vi "svx_Orbit Facade.vi"(0 "Data In":T5, 2 "Display State In":T3, 3 "Container State":T4) -> (6 "Data Out":T5, 7 "Display State Out":T3, 8 "Action":T2)   [LabVIEW 2017, in "SVX Orbit.xctl"]
uses:
  <vilib>/addons/_XControls/Orbit Plot/SVX Orbit.xctl
  <vilib>/addons/_XControls/Orbit Plot/subVIs/svx_Orbit Data.ctl
  <vilib>/_xctls/Container State.ctl
  <vilib>/addons/_XControls/Orbit Plot/subVIs/svx_Orbit State.ctl
  <vilib>/addons/_XControls/Orbit Plot/subVIs/svx_Orbit Internal State.ctl
  <vilib>/addons/_XControls/Orbit Plot/subVIs/svx_Orbit Bounds.ctl
  <vilib>/_xctls/Action.ctl
  <vilib>/Utility/miscctls.llb/LVPoint32TypeDef.ctl
  <vilib>/addons/_XControls/Orbit Plot/subVIs/svx_Orbit Core States.ctl
  <vilib>/_xctls/XControlSupport.lvlib
panel:
  out "Coords":T1
  out "Tree":string(tree)
  out "Cursor Info":string
  out "Orbit Plot":T6(graph)=[{"orbit plot X"=[1.0], "orbit plot Y"=[1.0]}, {"orbit plot X"=[0.0, 1.0], "orbit plot Y"=[1.0]}]
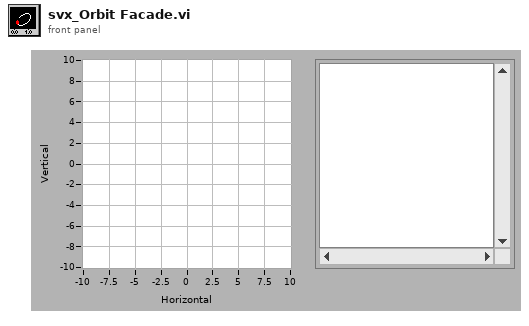
[diagram p1: front panel]
types:
  T1 = typedef "LVPoint32TypeDef.ctl" = cluster{"Horizontal":i32, "Vertical":i32}
  T2 = typedef "XControlSupport.lvlib/Action.ctl" = cluster{"Data Changed?":bool, "State Changed?":bool, "Action Name":string}
  T3 = typedef "SVX Orbit.xctl/svx_Orbit State.ctl" = cluster{"State Queue":refnum<queue>, "Old State":variant}
  T4 = typedef "XControlSupport.lvlib/Container State.ctl" = cluster{"Indicator?":bool, "Run Mode?":bool, " Refnum":refnum<vi>}
  T5 = typedef "SVX Orbit.xctl/svx_Orbit Data.ctl" = cluster{"probe x":dbl[], "probe y":dbl[], "reference":dbl[], "plot type":enum16{"Filtered Plot", "Unfiltered Plot"}, "attribute":variant}[][]
  T6 = cluster{"orbit plot X":dbl[], "orbit plot Y":dbl[]}[]
  T7 = cluster{"CursLoc.X":dbl, "Cursloc.Y":dbl, "PointIdx":i32}
  T8 = cluster{"Minimum":dbl, "Maximum":dbl, "Kind":enum16{"X-Scale", "Y-Scale", "Z-Scale"}}
  T9 = typedef "SVX Orbit.xctl/svx_Orbit Internal State.ctl" = cluster{"X Scale":cluster{"Name":string, "FString":string, "Major Color":u32, "Minor Color":u32, "Scale Visible":bool, " Label Visible":bool, "Grid Style":u16}, "Y Scale":cluster{"Name":string, "FString":string, "Major Color":u32, "Minor Color":u32, "Scale Visible":bool, " Label Visible":bool, "Grid Style":u16}, "Plot":cluster{"Point Style":u8, "Line Width":u8, "Line Style":u8, "Plot Color":u32, "Point/fill":u32}, "Arrow/Crosshair Color":u32, "Tacho Point Color":u32, "Container Bounds":T10, "Axis Maximum":dbl, "Probe Angles":cluster{"Angle X":dbl, "Angle Y":dbl}, "Background Color":u32, "Cursor":cluster{"Cursor Point Style":u8, "Cursor Style":u8, "Cursor Line Width":u8, "Cursor Line Style":u8, "Cursor Color":u32, "Cursor Name Visible":bool, "Cursor Visible":bool, "Cursor Position":cluster{"X":dbl, "Y":dbl}, "Cursor Index":i32, "Cursor Lock":bool}, "Elliptical Info":cluster{"a":dbl, "b":dbl, "e":dbl, "ang":dbl}[], "Legend Visible":bool, "Scale Range Change":refnum<user-event>, "Strings[]":cluster{"Custom pair name":bool, "Row Strings []":string[], "Column Strings []":string[]}, "Index":cluster{"pair index":i32, "order index":i32}[], " Parents Tags":string[], "Children Tags":string[], "Open?":bool[], "Label":string, "Legend Width":u32, "Pair Strings Changed?":bool, "Size":i32[], "Legend Background":u32, "Legend Font":u32, "Cursor Release":refnum<user-event>, "Autoscale":bool, "Precession Direction":enum16{"forward", "backward"}[], "Item Width":u32, "User Pair Strings []":string[], "Users Order Strings []":string[], "Autoscale Once":bool, "Property Write":refnum<queue>}
  T10 = typedef "SVX Orbit.xctl/svx_Orbit Bounds.ctl" = cluster{"Width":u32, "Height":u32}
  T11 = typedef "SVX Orbit.xctl/svx_Orbit Core States.ctl" = enum16{"None", "[Axis] Range", "[Plot] Image", "[Plot] Tacho Point", "[Plot] Grid and BG", "[Cursor] Cursor Info", "[Legend] Pair Strings", "[Data] Plot Data", "[Legend] Checkbox", "[Layout] Update", "[Legend] Tree Open", "[Layout] Legend Visible", "[Plot] Data Point", "[Axis] Axis and Label", "[Axis] Format String", "[Cursor] Appearance", "[Cursor] Index", "[Legend] Color", "[Layout] Min Pane Size", "[Data] Legend Strings"}
  T12 = typedef "LVRangeTypeDef.ctl" = cluster{"Minimum":dbl, "Maximum":dbl, "Increment":dbl, "Minor Increment":dbl, "Start":dbl}
  T13 = cluster{" Refnum":refnum<vi>, "Orbit Plot":refnum<vi>, "Tree":refnum<vi>, "Cursor Info":refnum<vi>, "This VI":refnum<vi>}
  T14 = cluster{"BG Color":u32, "XScale.MajGrdColor":u32, "XScale.MnrGrdColor":u32, "YScale.MajGrdColor":u32, "YScale.MnrGrdColor":u32}
  T15 = cluster{"Background Color":u32, "Major Color":u32, "Minor Color":u32, "Major Color":u32, "Minor Color":u32}
  T16 = typedef "LVRectTypeDef.ctl" = cluster{"Left":i16, "Top":i16, "Right":i16, "Bottom":i16}
  T17 = cluster{"Shift":bool, "Ctrl":bool, "Alt":bool, "Cmd":bool, "Opt":bool}
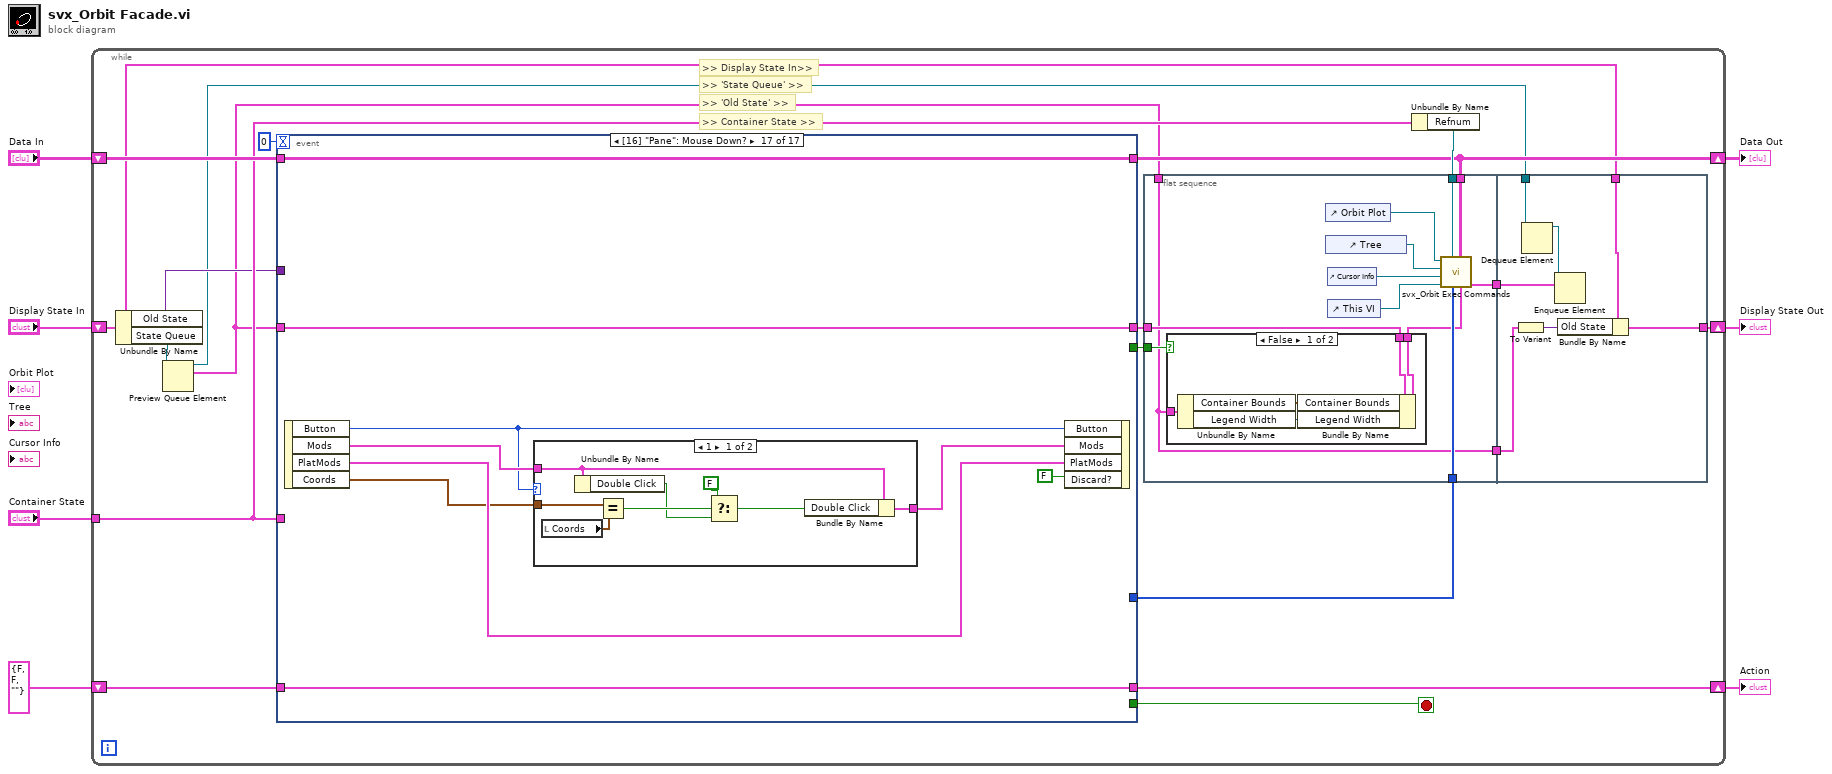
[diagram p0: block diagram]
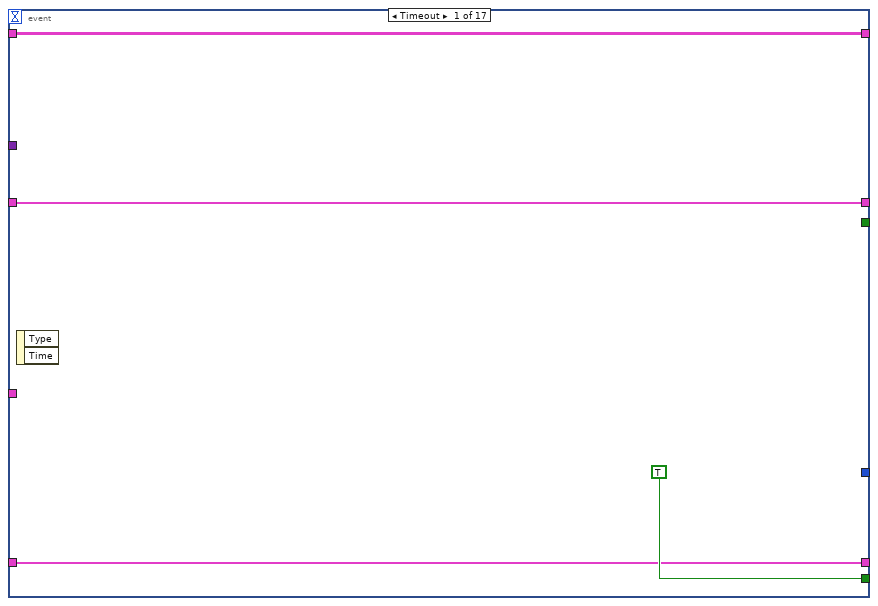
[diagram p3: hidden frame]
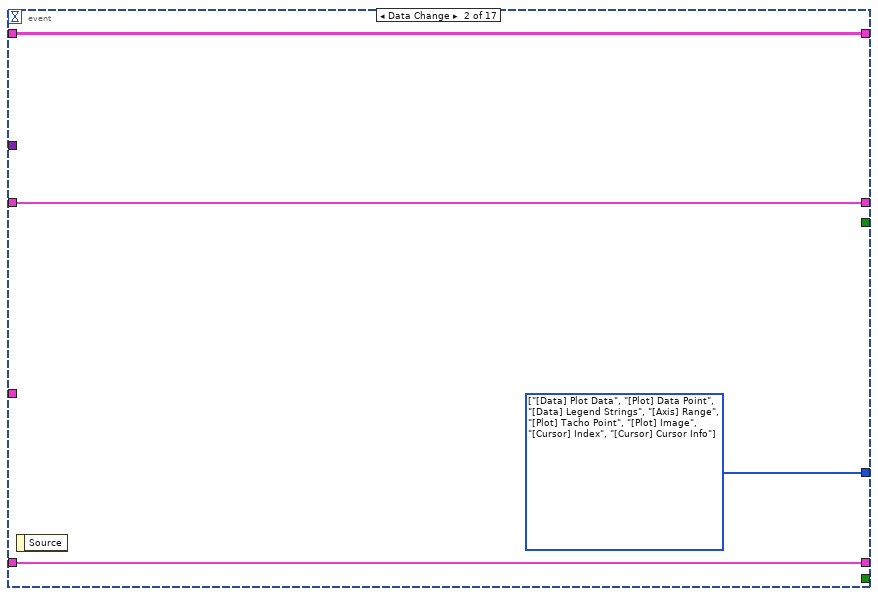
[diagram p4: hidden frame]
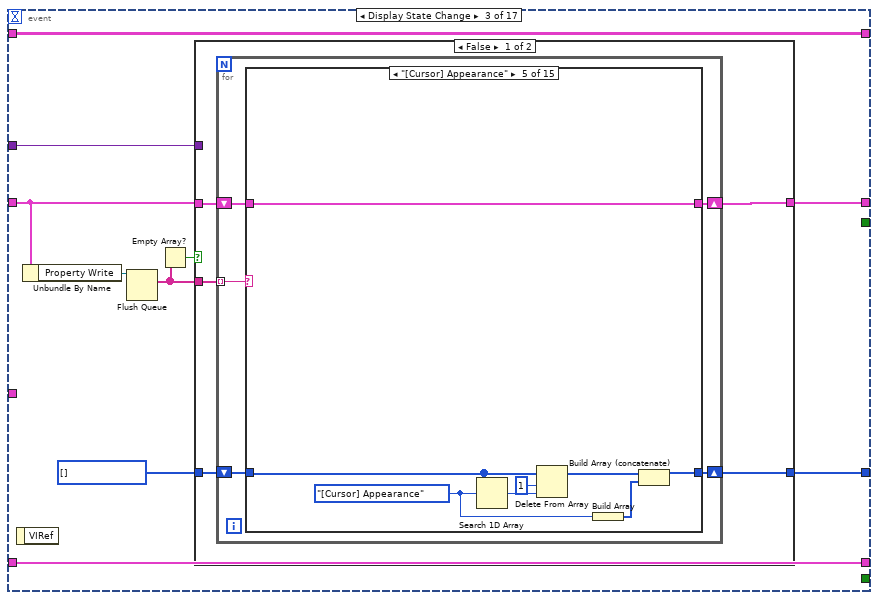
[diagram p5: hidden frame]
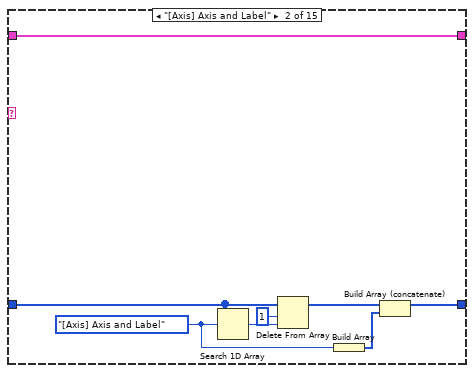
[diagram p7: hidden frame]
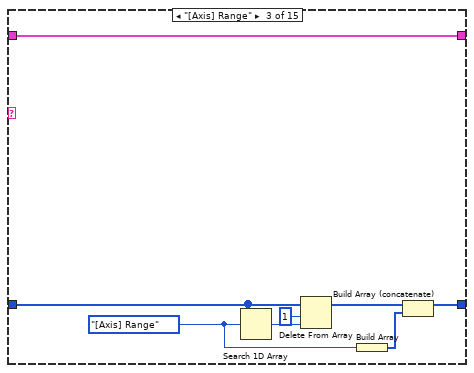
[diagram p8: hidden frame]
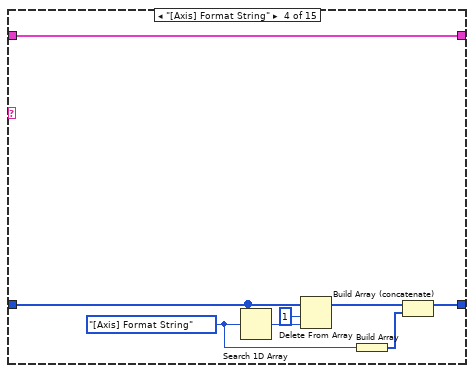
[diagram p9: hidden frame]
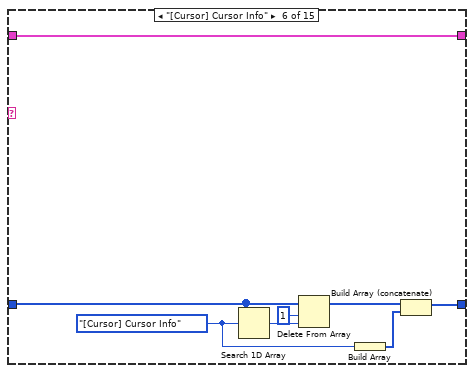
[diagram p10: hidden frame]
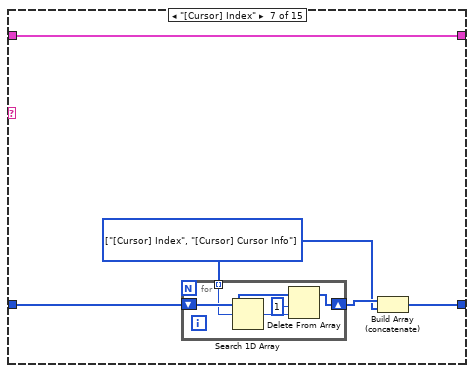
[diagram p11: hidden frame]
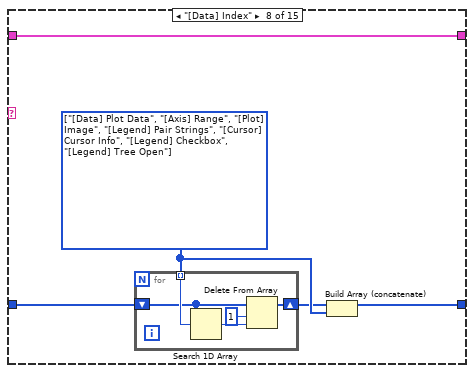
[diagram p12: hidden frame]
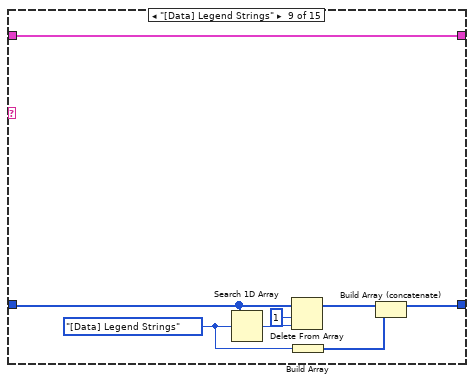
[diagram p13: hidden frame]
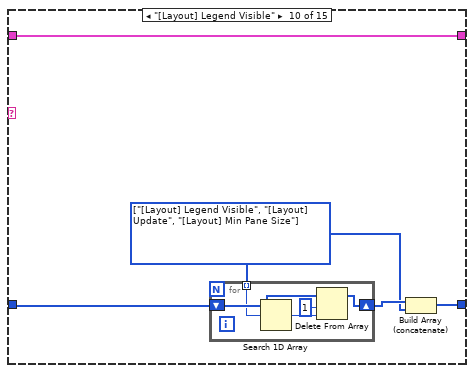
[diagram p14: hidden frame]
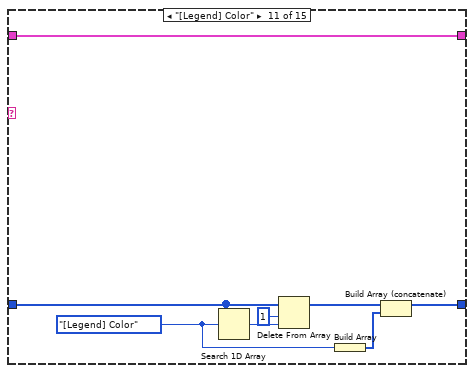
[diagram p15: hidden frame]
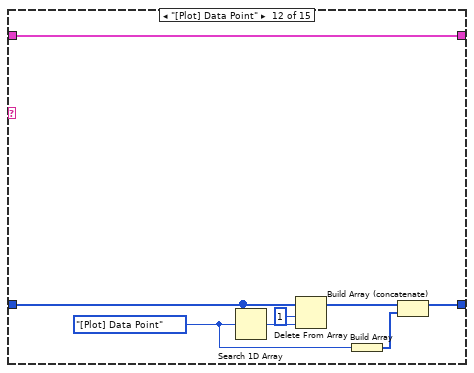
[diagram p16: hidden frame]
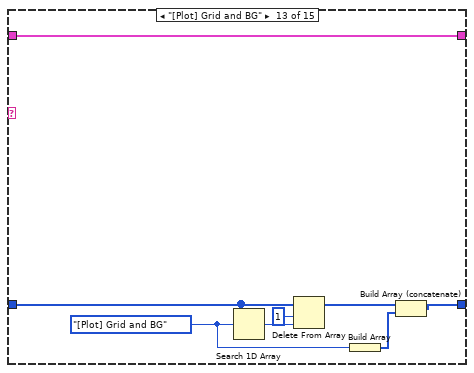
[diagram p17: hidden frame]
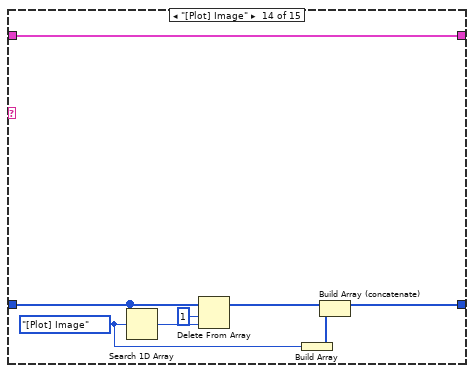
[diagram p18: hidden frame]
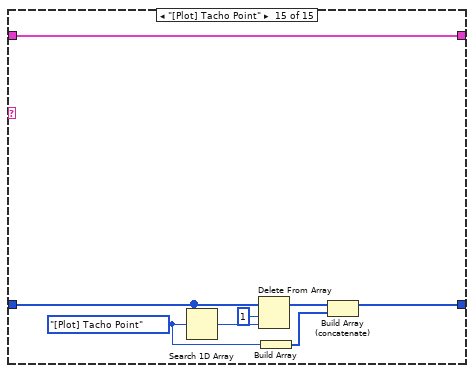
[diagram p19: hidden frame]
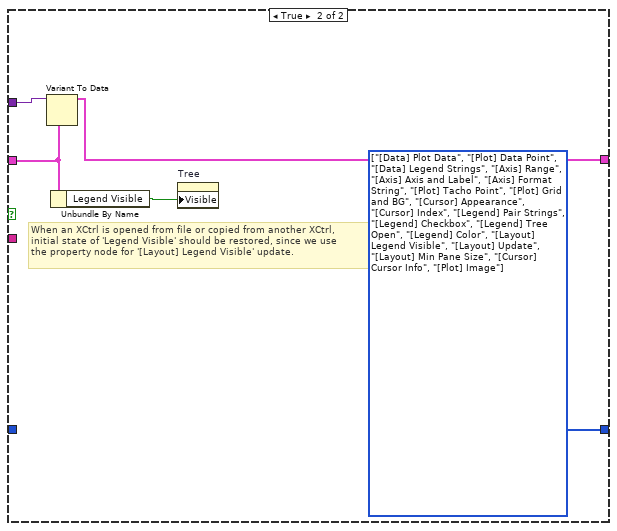
[diagram p20: hidden frame]
diagram:
  n1 = while {
    shift-right: [w11] -> w4
    shift-left: "Display State In" -> [w12]
    tunnel: "Container State" -> [w23]
    shift-right: [w21] -> w7
    shift-left: "Data In" -> [w25]
    shift-right: [w18] -> w2
    shift-left: T2 {"Data Changed?"=FALSE, "State Changed?"=FALSE, "Action Name"=""} ("Action") -> [w24]
    stop <- w16 stop-if-true
    # ">> Container State >>"
    # ">> 'Old State' >>"
    # ">> Display State In>>"
    # ">> 'State Queue' >>"
    n2 = Unbundle By Name(w12) -> ("Old State"=w15:variant, "State Queue"=w17:refnum<queue>)
    n3 = Preview Queue Element(queue=w17) -> (queue out=w13:refnum<queue>, element=w9:T9)  [unwired: 2 in, 2 out]
    n4 = event shown="[16] \"Pane\": Mouse Down?" {
      selector: _ -> [_ _ _ _ _ _ _ _ _ _ _ _ _ _ _ _ _]
      dyn-events: _ -> [_ _ _ _ _ _ _ _ _ _ _ _ _ _ _ _ _]
      timeout: 0 -> [_ _ _ _ _ _ _ _ _ _ _ _ _ _ _ _ _]
      tunnel: w9 -> [w52 w58 w60 w207 w210 w222 w256 w277 w288 w298 w397 w480 w510 w518 w557 w562 w581]
      tunnel: [w52 w58 w66 w207 w210 w214 w228 w280 w288 w297 w396 w479 w509 w521 w557 w562 w581] -> w20
      tunnel: [TRUE _ _ _ _ _ _ _ _ _ _ _ _ _ _ _ _] -> w16
      tunnel: w23 -> [_ _ _ _ _ _ _ _ w292 w303 _ _ _ _ _ _ _]
      tunnel: w25 -> [w54 w59 w65 w206 w209 w221 w261 w286 w294 w295 w400 w482 w504 w528 w555 w561 w582]
      tunnel: [w54 w59 w65 w206 w209 w221 w261 w286 w294 w295 w400 w481 w504 w528 w555 w561 w582] -> w21
      tunnel: [w53 w56 w64 w205 w208 w224 w259 w276 w293 w296 w394 w485 w507 w519 w556 w560 w580] -> w18
      tunnel: w24 -> [w53 w56 w64 w205 w208 w225 w260 w276 w293 w300 w395 w487 w508 w520 w556 w560 w580]
      tunnel: [_ w57 w68 _ _ w219 _ w285 _ w299 w393 w486 _ w517 _ _ _] -> w19
      tunnel: w15 -> [_ _ w63 _ _ _ _ _ _ _ _ _ _ _ _ _ _]
      tunnel: [_ _ _ _ _ _ _ TRUE _ _ _ _ _ _ _ _ _] -> w10
      event Timeout {
        n5 = event-data() -> ()  [unwired: 1 in, 2 out]
      }
      event Data Change {
        w57 = T11[] [enum."[Data] Plot Data", enum."[Plot] Data Point", enum."[Data] Legend Strings", enum."[Axis] Range", enum."[Plot] Tacho Point", enum."[Plot] Image", enum."[Cursor] Index", enum."[Cursor] Cursor Info"] items=["None", "[Axis] Range", "[Plot] Image", "[Plot] Tacho Point", "[Plot] Grid and BG", "[Cursor] Cursor Info", "[Legend] Pair Strings", "[Data] Plot Data", "[Legend] Checkbox", "[Layout] Update", "[Legend] Tree Open", "[Layout] Legend Visible", "[Plot] Data Point", "[Axis] Axis and Label", "[Axis] Format String", "[Cursor] Appearance", "[Cursor] Index", "[Legend] Color", "[Layout] Min Pane Size", "[Data] Legend Strings"] ("array")
        n6 = event-data() -> ()  [unwired: 1 in, 1 out]
      }
      event Display State Change {
        w67 = T11[] [] items=["None", "[Axis] Range", "[Plot] Image", "[Plot] Tacho Point", "[Plot] Grid and BG", "[Cursor] Cursor Info", "[Legend] Pair Strings", "[Data] Plot Data", "[Legend] Checkbox", "[Layout] Update", "[Legend] Tree Open", "[Layout] Legend Visible", "[Plot] Data Point", "[Axis] Axis and Label", "[Axis] Format String", "[Cursor] Appearance", "[Cursor] Index", "[Legend] Color", "[Layout] Min Pane Size", "[Data] Legend Strings"]
        n7 = event-data() -> ()  [unwired: 1 in, 1 out]
        n8 = Unbundle By Name(w60) -> ("Property Write"=w62:refnum<queue>)
        n9 = Flush Queue(queue=w62) -> (remaining elements=w61:string[])  [unwired: 1 in, 2 out]
        n10 = Empty Array?(array=w61) -> (empty?=w69:bool)
        n11 = case shown="False" w69 {
          tunnel: w60 -> [w72 w201]
          tunnel: [w73 w204] -> w68
          tunnel: w67 -> [w74 _]
          tunnel: [w71 w200] -> w66
          tunnel: w63 -> [_ w203]
          tunnel: w61 -> [w70 _]
          frame False {
            n12 = for {
              tunnel: w70 -> [w79] mode=indexing
              shift-right: [w77] -> w73
              shift-left: w74 -> [w78]
              shift-right: [w75] -> w71
              shift-left: w72 -> [w76]
              n13 = case shown="\"[Cursor] Appearance\"" w79 {
                tunnel: w78 -> [w81 w83 w91 w99 w107 w115 w124 w135 w144 w151 w161 w169 w178 w187 w195]
                tunnel: [w81 w82 w90 w98 w106 w114 w123 w132 w143 w150 w160 w168 w177 w191 w199] -> w77
                tunnel: w76 -> [w80 w89 w97 w105 w113 w121 w126 w136 w149 w154 w167 w175 w183 w190 w198]
                tunnel: [w80 w89 w97 w105 w113 w121 w126 w136 w149 w154 w167 w175 w183 w190 w198] -> w75
                frame "", Default {
                }
                frame "[Axis] Axis and Label" {
                  w84 = svx_Orbit_Core_States."[Axis] Axis and Label" ("Property Page User Events")
                  n14 = Search 1D Array(1D array=w83, element=w84) -> (index of element=w88:i32)  [unwired: 1 in]
                  n15 = Delete From Array(array=w83, length=1, index=w88) -> (array with subset deleted=w86:T11[])  [unwired: 1 out]
                  n16 = Build Array(w84) -> (w85:T11[])
                  n17 = Build Array (concatenate)(w86, w85) -> (w82:T11[])
                }
                frame "[Axis] Range" {
                  w92 = svx_Orbit_Core_States."[Axis] Range" ("Property Page User Events")
                  n18 = Search 1D Array(1D array=w91, element=w92) -> (index of element=w96:i32)  [unwired: 1 in]
                  n19 = Delete From Array(array=w91, length=1, index=w96) -> (array with subset deleted=w94:T11[])  [unwired: 1 out]
                  n20 = Build Array(w92) -> (w93:T11[])
                  n21 = Build Array (concatenate)(w94, w93) -> (w90:T11[])
                }
                frame "[Axis] Format String" {
                  w100 = svx_Orbit_Core_States."[Axis] Format String" ("Property Page User Events")
                  n22 = Search 1D Array(1D array=w99, element=w100) -> (index of element=w104:i32)  [unwired: 1 in]
                  n23 = Delete From Array(array=w99, length=1, index=w104) -> (array with subset deleted=w102:T11[])  [unwired: 1 out]
                  n24 = Build Array(w100) -> (w101:T11[])
                  n25 = Build Array (concatenate)(w102, w101) -> (w98:T11[])
                }
                frame "[Cursor] Appearance" {
                  w109 = svx_Orbit_Core_States."[Cursor] Appearance" ("Property Page User Events")
                  n26 = Search 1D Array(1D array=w107, element=w109) -> (index of element=w112:i32)  [unwired: 1 in]
                  n27 = Delete From Array(array=w107, length=1, index=w112) -> (array with subset deleted=w108:T11[])  [unwired: 1 out]
                  n28 = Build Array(w109) -> (w110:T11[])
                  n29 = Build Array (concatenate)(w108, w110) -> (w106:T11[])
                }
                frame "[Cursor] Cursor Info" {
                  w117 = svx_Orbit_Core_States."[Cursor] Cursor Info" ("Property Page User Events")
                  n30 = Search 1D Array(1D array=w115, element=w117) -> (index of element=w120:i32)  [unwired: 1 in]
                  n31 = Delete From Array(array=w115, length=1, index=w120) -> (array with subset deleted=w116:T11[])  [unwired: 1 out]
                  n32 = Build Array(w117) -> (w118:T11[])
                  n33 = Build Array (concatenate)(w116, w118) -> (w114:T11[])
                }
                frame "[Cursor] Index" {
                  w122 = T11[] [enum."[Cursor] Index", enum."[Cursor] Cursor Info"] items=["None", "[Axis] Range", "[Plot] Image", "[Plot] Tacho Point", "[Plot] Grid and BG", "[Cursor] Cursor Info", "[Legend] Pair Strings", "[Data] Plot Data", "[Legend] Checkbox", "[Layout] Update", "[Legend] Tree Open", "[Layout] Legend Visible", "[Plot] Data Point", "[Axis] Axis and Label", "[Axis] Format String", "[Cursor] Appearance", "[Cursor] Index", "[Legend] Color", "[Layout] Min Pane Size", "[Data] Legend Strings"]
                  n34 = for {
                    shift-right: [w128] -> w125
                    shift-left: w124 -> [w129]
                    tunnel: w122 -> [w127] mode=indexing
                    n35 = Search 1D Array(1D array=w129, element=w127) -> (index of element=w131:i32)  [unwired: 1 in]
                    n36 = Delete From Array(array=w129, length=1, index=w131) -> (array with subset deleted=w128:T11[])  [unwired: 1 out]
                  }
                  n37 = Build Array (concatenate)(w125, w122) -> (w123:T11[])
                }
                frame "[Data] Index" {
                  w134 = T11[] [enum."[Data] Plot Data", enum."[Axis] Range", enum."[Plot] Image", enum."[Legend] Pair Strings", enum."[Cursor] Cursor Info", enum."[Legend] Checkbox", enum."[Legend] Tree Open"] items=["None", "[Axis] Range", "[Plot] Image", "[Plot] Tacho Point", "[Plot] Grid and BG", "[Cursor] Cursor Info", "[Legend] Pair Strings", "[Data] Plot Data", "[Legend] Checkbox", "[Layout] Update", "[Legend] Tree Open", "[Layout] Legend Visible", "[Plot] Data Point", "[Axis] Axis and Label", "[Axis] Format String", "[Cursor] Appearance", "[Cursor] Index", "[Legend] Color", "[Layout] Min Pane Size", "[Data] Legend Strings"]
                  n38 = for {
                    tunnel: w134 -> [w139] mode=indexing
                    shift-right: [w137] -> w133
                    shift-left: w135 -> [w138]
                    n39 = Search 1D Array(1D array=w138, element=w139) -> (index of element=w141:i32)  [unwired: 1 in]
                    n40 = Delete From Array(array=w138, length=1, index=w141) -> (array with subset deleted=w137:T11[])  [unwired: 1 out]
                  }
                  n41 = Build Array (concatenate)(w133, w134) -> (w132:T11[])
                }
                frame "[Data] Legend Strings" {
                  w142 = svx_Orbit_Core_States."[Data] Legend Strings" ("Property Page User Events")
                  n42 = Search 1D Array(1D array=w144, element=w142) -> (index of element=w148:i32)  [unwired: 1 in]
                  n43 = Delete From Array(array=w144, length=1, index=w148) -> (array with subset deleted=w146:T11[])  [unwired: 1 out]
                  n44 = Build Array(w142) -> (w145:T11[])
                  n45 = Build Array (concatenate)(w146, w145) -> (w143:T11[])
                }
                frame "[Layout] Legend Visible" {
                  w152 = T11[] [enum."[Layout] Legend Visible", enum."[Layout] Update", enum."[Layout] Min Pane Size"] items=["None", "[Axis] Range", "[Plot] Image", "[Plot] Tacho Point", "[Plot] Grid and BG", "[Cursor] Cursor Info", "[Legend] Pair Strings", "[Data] Plot Data", "[Legend] Checkbox", "[Layout] Update", "[Legend] Tree Open", "[Layout] Legend Visible", "[Plot] Data Point", "[Axis] Axis and Label", "[Axis] Format String", "[Cursor] Appearance", "[Cursor] Index", "[Legend] Color", "[Layout] Min Pane Size", "[Data] Legend Strings"]
                  n46 = for {
                    shift-right: [w156] -> w153
                    shift-left: w151 -> [w157]
                    tunnel: w152 -> [w155] mode=indexing
                    n47 = Search 1D Array(1D array=w157, element=w155) -> (index of element=w159:i32)  [unwired: 1 in]
                    n48 = Delete From Array(array=w157, length=1, index=w159) -> (array with subset deleted=w156:T11[])  [unwired: 1 out]
                  }
                  n49 = Build Array (concatenate)(w153, w152) -> (w150:T11[])
                }
                frame "[Legend] Color" {
                  w162 = svx_Orbit_Core_States."[Legend] Color" ("Property Page User Events")
                  n50 = Search 1D Array(1D array=w161, element=w162) -> (index of element=w166:i32)  [unwired: 1 in]
                  n51 = Delete From Array(array=w161, length=1, index=w166) -> (array with subset deleted=w164:T11[])  [unwired: 1 out]
                  n52 = Build Array(w162) -> (w163:T11[])
                  n53 = Build Array (concatenate)(w164, w163) -> (w160:T11[])
                }
                frame "[Plot] Data Point" {
                  w171 = svx_Orbit_Core_States."[Plot] Data Point" ("Property Page User Events")
                  n54 = Search 1D Array(1D array=w169, element=w171) -> (index of element=w174:i32)  [unwired: 1 in]
                  n55 = Delete From Array(array=w169, length=1, index=w174) -> (array with subset deleted=w170:T11[])  [unwired: 1 out]
                  n56 = Build Array(w171) -> (w172:T11[])
                  n57 = Build Array (concatenate)(w170, w172) -> (w168:T11[])
                }
                frame "[Plot] Grid and BG" {
                  w179 = svx_Orbit_Core_States."[Plot] Grid and BG" ("Property Page User Events")
                  n58 = Search 1D Array(1D array=w178, element=w179) -> (index of element=w182:i32)  [unwired: 1 in]
                  n59 = Delete From Array(array=w178, length=1, index=w182) -> (array with subset deleted=w176:T11[])  [unwired: 1 out]
                  n60 = Build Array(w179) -> (w180:T11[])
                  n61 = Build Array (concatenate)(w176, w180) -> (w177:T11[])
                }
                frame "[Plot] Image" {
                  w185 = svx_Orbit_Core_States."[Plot] Image" ("Property Page User Events")
                  n62 = Search 1D Array(1D array=w187, element=w185) -> (index of element=w189:i32)  [unwired: 1 in]
                  n63 = Delete From Array(array=w187, length=1, index=w189) -> (array with subset deleted=w186:T11[])  [unwired: 1 out]
                  n64 = Build Array(w185) -> (w184:T11[])
                  n65 = Build Array (concatenate)(w186, w184) -> (w191:T11[])
                }
                frame "[Plot] Tacho Point" {
                  w193 = svx_Orbit_Core_States."[Plot] Tacho Point" ("Property Page User Events")
                  n66 = Search 1D Array(1D array=w195, element=w193) -> (index of element=w197:i32)  [unwired: 1 in]
                  n67 = Delete From Array(array=w195, length=1, index=w197) -> (array with subset deleted=w194:T11[])  [unwired: 1 out]
                  n68 = Build Array(w193) -> (w192:T11[])
                  n69 = Build Array (concatenate)(w194, w192) -> (w199:T11[])
                }
              }
            }
          }
          frame True {
            w204 = T11[] [enum."[Data] Plot Data", enum."[Plot] Data Point", enum."[Data] Legend Strings", enum."[Axis] Range", enum."[Axis] Axis and Label", enum."[Axis] Format String", enum."[Plot] Tacho Point", enum."[Plot] Grid and BG", enum."[Cursor] Appearance", enum."[Cursor] Index", enum."[Legend] Pair Strings", enum."[Legend] Checkbox", enum."[Legend] Tree Open", enum."[Legend] Color", enum."[Layout] Legend Visible", enum."[Layout] Update", enum."[Layout] Min Pane Size", enum."[Cursor] Cursor Info", enum."[Plot] Image"] items=["None", "[Axis] Range", "[Plot] Image", "[Plot] Tacho Point", "[Plot] Grid and BG", "[Cursor] Cursor Info", "[Legend] Pair Strings", "[Data] Plot Data", "[Legend] Checkbox", "[Layout] Update", "[Legend] Tree Open", "[Layout] Legend Visible", "[Plot] Data Point", "[Axis] Axis and Label", "[Axis] Format String", "[Cursor] Appearance", "[Cursor] Index", "[Legend] Color", "[Layout] Min Pane Size", "[Data] Legend Strings"]
            # "When an XCtrl is opened from file or copied from another XCtrl,\ninitial state of 'Legend Visible' should be restored, since we use\nthe property node for '[Layout] Legend Visible' update."
            n70 = Variant To Data(type=w201, Variant=w203) -> (data=w200:T9)  [unwired: 1 in, 1 out]
            n71 = Unbundle By Name(w201) -> ("Legend Visible"=w202:bool)
            n72 = property on="Tree" class="Tree (strict)"("Visible"=w202) -> ()  [unwired: 2 in, 2 out]
          }
        }
      }
      event Direction Change {
        n73 = event-data() -> ()  [unwired: 1 in, 4 out]
      }
      event Exec State Change {
        n74 = event-data() -> ()  [unwired: 1 in, 4 out]
      }
      event "Orbit Plot": Cursor Release {
        w219 = T11[] [enum."[Cursor] Cursor Info"] items=["None", "[Axis] Range", "[Plot] Image", "[Plot] Tacho Point", "[Plot] Grid and BG", "[Cursor] Cursor Info", "[Legend] Pair Strings", "[Data] Plot Data", "[Legend] Checkbox", "[Layout] Update", "[Legend] Tree Open", "[Layout] Legend Visible", "[Plot] Data Point", "[Axis] Axis and Label", "[Axis] Format String", "[Cursor] Appearance", "[Cursor] Index", "[Legend] Color", "[Layout] Min Pane Size", "[Data] Legend Strings"] ("f")
        n75 = event-data() -> ("CursLoc"=w218:cluster{"X":dbl, "Y":dbl}, "PointIdx"=w212:i32)  [unwired: 1 in]
        n76 = Unbundle By Name(w218) -> ("X"=w217:dbl, "Y"=w216:dbl)
        n77 = Bundle By Name(cluster=w222, "Cursor.Cursor Position"=w218, "Cursor.Cursor Index"=w212) -> (w214:T9)
        n78 = Bundle By Name(cluster=T7 {"CursLoc.X"=0.0, "Cursloc.Y"=0.0, "PointIdx"=0} ("event data"), "CursLoc.X"=w217, "Cursloc.Y"=w216, "PointIdx"=w212) -> (w211:T7)
        n79 = Bundle By Name(cluster=w225, "State Changed?"=TRUE, "Action Name"="Move") -> (w224:T2)
        n80 = Unbundle By Name(w214) -> ("Cursor Release"=w215:refnum<user-event>)
        n81 = Generate User Event(user event=w215, event data cluster=w211) -> ()  [unwired: 2 in, 2 out]
      }
      event "Orbit Plot": Scale Range Change {
        n82 = event-data() -> ("NewRange.Maximum"=w254:dbl, "NewRange.Minimum"=w253:dbl, "Kind"=w233:enum16{"X-Scale", "Y-Scale", "Z-Scale"})  [unwired: 1 in]
        n83 = property on="Orbit Plot" class="XYGraph (strict)"() -> ("YScale.Range"=w251:T12, "XScale.Range"=w250:T12)  [unwired: 2 in, 2 out]
        n84 = Unbundle By Name(w256) -> ("Axis Maximum"=w243:dbl)
        n85 = Unbundle By Name(w251) -> ("Minimum"=w249:dbl, "Maximum"=w246:dbl)
        n86 = Unbundle By Name(w250) -> ("Minimum"=w248:dbl, "Maximum"=w244:dbl)
        n87 = Absolute Value(x=w248) -> (abs(x)=w245:dbl)
        n88 = Absolute Value(x=w249) -> (abs(x)=w247:dbl)
        n89 = Not Equal?(x=w243, y=w254) -> (x != y?=w255:bool)
        n90 = Build Array(w247, w246, w245, w244) -> (w242:dbl[])
        n91 = Not Equal?(x=w242, y=w243) -> (x != y?=w239:bool[])
        n92 = Select(t=w254, s=w255, f=w253) -> (s? t:f=w252:dbl)
        n93 = And Array Elements(Boolean array=w239) -> (logical AND=w237:bool)
        n94 = Or Array Elements(Boolean array=w239) -> (logical OR=w238:bool)
        n95 = Array Max & Min(array=w242) -> (max value=w241:dbl)  [unwired: 3 out]
        n96 = Absolute Value(x=w252) -> (abs(x)=w240:dbl)
        n97 = Not(x=w238) -> (.not. x?=w236:bool)
        n98 = Or(x=w237, y=w236) -> (x .or. y?=w235:bool)
        n99 = Select(t=w241, s=w235, f=w240) -> (s? t:f=w230:dbl)
        n100 = Bundle By Name(cluster=w260, "Action Name"="Range Changed", "State Changed?"=TRUE) -> (w259:T2)
        n101 = Negate(x=w230) -> (-x=w231:dbl)
        n102 = case shown="\"X-Scale\", Default" w233 {
          tunnel: w231 -> [w263 w270]
          tunnel: w230 -> [w262 w269]
          tunnel: FALSE ("X Scale.Flipped") -> [w264 w268]
          frame "X-Scale", Default {
            n103 = property on="Orbit Plot" class="XYGraph (strict)"("XScale.Minimum"=w263, "XScale.Maximum"=w262, "XScale.Flipped"=w264) -> (error out=w267:errorcluster)  [unwired: 2 in, 1 out]
            n104 = property on="Orbit Plot" class="XYGraph (strict)"(error in=w267) -> (error out=w266:errorcluster, "XScale.Range"=w265:T12)  [unwired: 1 in, 1 out]
            n105 = property on="Orbit Plot" class="XYGraph (strict)"(error in=w266, "YScale.Range"=w265) -> ()  [unwired: 1 in, 2 out]
          }
          frame "Y-Scale" {
            n106 = property on="Orbit Plot" class="XYGraph (strict)"("YScale.Minimum"=w270, "YScale.Maximum"=w269, "YScale.Flipped"=w268) -> (error out=w273:errorcluster)  [unwired: 2 in, 1 out]
            n107 = property on="Orbit Plot" class="XYGraph (strict)"(error in=w273) -> (error out=w272:errorcluster, "YScale.Range"=w271:T12)  [unwired: 1 in, 1 out]
            n108 = property on="Orbit Plot" class="XYGraph (strict)"(error in=w272, "XScale.Range"=w271) -> ()  [unwired: 1 in, 2 out]
          }
        }
        n109 = Bundle By Name(cluster=w256, "Autoscale"=FALSE ("autoscale"), "Axis Maximum"=w230) -> (w228:T9)
        n110 = Bundle By Name(cluster=T8 {"Minimum"=0.0, "Maximum"=0.0, "Kind"=enum."X-Scale"} ("output cluster"), "Minimum"=w231, "Maximum"=w230, "Kind"=w233) -> (w227:T8)
        n111 = Unbundle By Name(w228) -> ("Scale Range Change"=w229:refnum<user-event>)
        n112 = Generate User Event(user event=w229, event data cluster=w227) -> ()  [unwired: 2 in, 2 out]
      }
      event Pane Size {
        w285 = T11[] [enum."[Layout] Update", enum."[Plot] Image", enum."[Cursor] Cursor Info"] items=["None", "[Axis] Range", "[Plot] Image", "[Plot] Tacho Point", "[Plot] Grid and BG", "[Cursor] Cursor Info", "[Legend] Pair Strings", "[Data] Plot Data", "[Legend] Checkbox", "[Layout] Update", "[Legend] Tree Open", "[Layout] Legend Visible", "[Plot] Data Point", "[Axis] Axis and Label", "[Axis] Format String", "[Cursor] Appearance", "[Cursor] Index", "[Legend] Color", "[Layout] Min Pane Size", "[Data] Legend Strings"] ("f")
        n113 = event-data() -> ("NewBnds.Right"=w284:i16, "NewBnds.Left"=w283:i16, "NewBnds.Bottom"=w282:i16, "NewBnds.Top"=w281:i16)  [unwired: 1 in]
        n114 = Subtract(x=w284, y=w283) -> (x-y=w279:i16)
        n115 = Subtract(x=w282, y=w281) -> (x-y=w278:i16)
        n116 = Bundle(w279, w278) -> (w275:cluster{i16, i16})  [unwired: 1 in]
        n117 = Bundle By Name(cluster=w277, "Container Bounds"=w275) -> (w280:T9)
      }
      event "Orbit Plot": Shortcut Menu Activation? {
        n118 = event-data() -> ("Coords"=→"Coords":T1, "MenuRef"=w291:refnum<k9>)  [unwired: 1 in]
        n119 = Unbundle By Name(w292) -> ("Refnum"=w290:refnum<vi>, "Run Mode?"=w289:bool)
        n120 = call <vilib>:"svx_Orbit SC Menu.vi"("Run Mode?"=w289, "State"=w288, "Refnum"=w290, "MenuRef"=w291) -> ()  [unwired: 8 in]
        n121 = event-data() -> ()  [unwired: 2 in, 1 out]
      }
      event "Orbit Plot": Shortcut Menu Selection (User) {
        n122 = event-data() -> ("ItemTag"=w302:string)  [unwired: 1 in]
        n123 = Unbundle By Name(w303) -> ("Refnum"=w301:refnum<vi>)
        n124 = case shown="\"USER_SC_Y_SCALE\"" w302 {
          tunnel: w301 -> [_ w311 w317 _ _ _ _ _ _ w374 _]
          tunnel: w300 -> [w305 w307 w313 w325 w334 w338 w347 w357 w366 w380 w390]
          tunnel: [_ _ _ w318 w327 w341 w350 w355 w363 _ w391] -> w299
          tunnel: w298 -> [w304 w306 w312 w320 w329 w344 w353 w362 w371 w382 w387]
          tunnel: [w304 w306 w312 w326 w335 w343 w352 w361 w370 w381 w386] -> w297
          tunnel: [w305 w307 w313 w324 w333 w337 w346 w356 w365 w379 w389] -> w296
          tunnel: w295 -> [_ _ _ _ _ _ _ _ _ w373 _]
          frame "False", Default {
          }
          frame "USER_SC_LABEL" {
            n125 = property class="Ctl"(reference=w311) -> (reference out=w308:refnum<vi>, "Label.Visible"=w310:bool)  [unwired: 1 in, 1 out]
            n126 = Not(x=w310) -> (.not. x?=w309:bool)
            n127 = property class="Ctl"(reference=w308, "Label.Visible"=w309) -> ()  [unwired: 1 in, 2 out]
          }
          frame "USER_SC_CAPTION" {
            n128 = property class="Ctl"(reference=w317) -> (reference out=w314:refnum<vi>, "Caption.Visible"=w316:bool)  [unwired: 1 in, 1 out]
            n129 = Not(x=w316) -> (.not. x?=w315:bool)
            n130 = property class="Ctl"(reference=w314, "Caption.Visible"=w315) -> ()  [unwired: 1 in, 2 out]
          }
          frame "USER_SC_X_SCALE" {
            w318 = T11[] [enum."[Axis] Axis and Label"] items=["None", "[Axis] Range", "[Plot] Image", "[Plot] Tacho Point", "[Plot] Grid and BG", "[Cursor] Cursor Info", "[Legend] Pair Strings", "[Data] Plot Data", "[Legend] Checkbox", "[Layout] Update", "[Legend] Tree Open", "[Layout] Legend Visible", "[Plot] Data Point", "[Axis] Axis and Label", "[Axis] Format String", "[Cursor] Appearance", "[Cursor] Index", "[Legend] Color", "[Layout] Min Pane Size", "[Data] Legend Strings"] ("f")
            n131 = Unbundle By Name(w320) -> ("X Scale.Scale Visible"=w319:bool)
            n132 = Bundle By Name(cluster=w325, "Action Name"="Show/Hide", "State Changed?"=TRUE) -> (w324:T2)
            n133 = Not(x=w319) -> (.not. x?=w321:bool)
            n134 = Bundle By Name(cluster=w320, "X Scale.Scale Visible"=w321) -> (w326:T9)
          }
          frame "USER_SC_Y_SCALE" {
            w327 = T11[] [enum."[Axis] Axis and Label"] items=["None", "[Axis] Range", "[Plot] Image", "[Plot] Tacho Point", "[Plot] Grid and BG", "[Cursor] Cursor Info", "[Legend] Pair Strings", "[Data] Plot Data", "[Legend] Checkbox", "[Layout] Update", "[Legend] Tree Open", "[Layout] Legend Visible", "[Plot] Data Point", "[Axis] Axis and Label", "[Axis] Format String", "[Cursor] Appearance", "[Cursor] Index", "[Legend] Color", "[Layout] Min Pane Size", "[Data] Legend Strings"] ("f")
            n135 = Unbundle By Name(w329) -> ("Y Scale.Scale Visible"=w328:bool)
            n136 = Bundle By Name(cluster=w334, "Action Name"="Show/Hide", "State Changed?"=TRUE) -> (w333:T2)
            n137 = Not(x=w328) -> (.not. x?=w330:bool)
            n138 = Bundle By Name(cluster=w329, "Y Scale.Scale Visible"=w330) -> (w335:T9)
          }
          frame "USER_SC_CURSOR" {
            w341 = T11[] [enum."[Cursor] Cursor Info"] items=["None", "[Axis] Range", "[Plot] Image", "[Plot] Tacho Point", "[Plot] Grid and BG", "[Cursor] Cursor Info", "[Legend] Pair Strings", "[Data] Plot Data", "[Legend] Checkbox", "[Layout] Update", "[Legend] Tree Open", "[Layout] Legend Visible", "[Plot] Data Point", "[Axis] Axis and Label", "[Axis] Format String", "[Cursor] Appearance", "[Cursor] Index", "[Legend] Color", "[Layout] Min Pane Size", "[Data] Legend Strings"] ("f")
            n139 = Unbundle By Name(w344) -> ("Cursor.Cursor Visible"=w342:bool)
            n140 = Bundle By Name(cluster=w338, "Action Name"="Show/Hide", "State Changed?"=TRUE) -> (w337:T2)
            n141 = Not(x=w342) -> (.not. x?=w336:bool)
            n142 = Bundle By Name(cluster=w344, "Cursor.Cursor Visible"=w336) -> (w343:T9)
          }
          frame "USER_SC_CURSORINFO" {
            w350 = T11[] [enum."[Cursor] Cursor Info"] items=["None", "[Axis] Range", "[Plot] Image", "[Plot] Tacho Point", "[Plot] Grid and BG", "[Cursor] Cursor Info", "[Legend] Pair Strings", "[Data] Plot Data", "[Legend] Checkbox", "[Layout] Update", "[Legend] Tree Open", "[Layout] Legend Visible", "[Plot] Data Point", "[Axis] Axis and Label", "[Axis] Format String", "[Cursor] Appearance", "[Cursor] Index", "[Legend] Color", "[Layout] Min Pane Size", "[Data] Legend Strings"] ("f")
            n143 = Unbundle By Name(w353) -> ("Cursor.Cursor Name Visible"=w351:bool)
            n144 = Bundle By Name(cluster=w347, "Action Name"="Show/Hide", "State Changed?"=TRUE) -> (w346:T2)
            n145 = Not(x=w351) -> (.not. x?=w345:bool)
            n146 = Bundle By Name(cluster=w353, "Cursor.Cursor Name Visible"=w345) -> (w352:T9)
          }
          frame "USER_SC_SELECTOR" {
            w355 = T11[] [enum."[Layout] Legend Visible", enum."[Layout] Update", enum."[Layout] Min Pane Size"] items=["None", "[Axis] Range", "[Plot] Image", "[Plot] Tacho Point", "[Plot] Grid and BG", "[Cursor] Cursor Info", "[Legend] Pair Strings", "[Data] Plot Data", "[Legend] Checkbox", "[Layout] Update", "[Legend] Tree Open", "[Layout] Legend Visible", "[Plot] Data Point", "[Axis] Axis and Label", "[Axis] Format String", "[Cursor] Appearance", "[Cursor] Index", "[Legend] Color", "[Layout] Min Pane Size", "[Data] Legend Strings"] ("f")
            n147 = Unbundle By Name(w362) -> ("Legend Visible"=w360:bool)
            n148 = Bundle By Name(cluster=w357, "Action Name"="Show Selector", "State Changed?"=TRUE) -> (w356:T2)
            n149 = Not(x=w360) -> (.not. x?=w354:bool)
            n150 = Bundle By Name(cluster=w362, "Legend Visible"=w354) -> (w361:T9)
          }
          frame "USER_SC_LOCK" {
            w363 = T11[] [enum."[Cursor] Cursor Info"] items=["None", "[Axis] Range", "[Plot] Image", "[Plot] Tacho Point", "[Plot] Grid and BG", "[Cursor] Cursor Info", "[Legend] Pair Strings", "[Data] Plot Data", "[Legend] Checkbox", "[Layout] Update", "[Legend] Tree Open", "[Layout] Legend Visible", "[Plot] Data Point", "[Axis] Axis and Label", "[Axis] Format String", "[Cursor] Appearance", "[Cursor] Index", "[Legend] Color", "[Layout] Min Pane Size", "[Data] Legend Strings"] ("f")
            n151 = Unbundle By Name(w371) -> ("Cursor.Cursor Lock"=w369:bool)
            n152 = Bundle By Name(cluster=w366, "Action Name"="Lock Cursor", "State Changed?"=TRUE) -> (w365:T2)
            n153 = Not(x=w369) -> (.not. x?=w364:bool)
            n154 = Bundle By Name(cluster=w371, "Cursor.Cursor Lock"=w364) -> (w370:T9)
          }
          frame "USER_SC_PROPERTIES" {
            n155 = control-ref of="Orbit Plot"() -> (w378:refnum<vi>)
            n156 = control-ref of="Tree"() -> (w377:refnum<vi>)
            n157 = control-ref of="Cursor Info"() -> (w376:refnum<vi>)
            n158 = control-ref of="This VI"() -> (w375:refnum<vi>)
            n159 = Bundle("Refnum"=w374, "Orbit Plot"=w378, "Tree"=w377, "Cursor Info"=w376, "This VI"=w375) -> (w372:T13)  [unwired: 1 in]
            n160 = call <vilib>:"svx_Orbit Property Dialog.vi"("Action in"=w380, "State in"=w382, "Ref In"=w372, "Orbit Plot"=w373) -> ("Action out"=w379:T2, "State out"=w381:T9)  [unwired: 6 in]
          }
          frame "USER_SC_AUTOSCALE" {
            w391 = T11[] [enum."[Axis] Range"] items=["None", "[Axis] Range", "[Plot] Image", "[Plot] Tacho Point", "[Plot] Grid and BG", "[Cursor] Cursor Info", "[Legend] Pair Strings", "[Data] Plot Data", "[Legend] Checkbox", "[Layout] Update", "[Legend] Tree Open", "[Layout] Legend Visible", "[Plot] Data Point", "[Axis] Axis and Label", "[Axis] Format String", "[Cursor] Appearance", "[Cursor] Index", "[Legend] Color", "[Layout] Min Pane Size", "[Data] Legend Strings"] ("f")
            n161 = Unbundle By Name(w387) -> ("Autoscale"=w384:bool)
            n162 = Bundle By Name(cluster=w390, "Action Name"="Graph Scale Option", "State Changed?"=TRUE) -> (w389:T2)
            n163 = Not(x=w384) -> (.not. x?=w383:bool)
            n164 = Bundle By Name(cluster=w387, "Autoscale"=w383) -> (w386:T9)
          }
        }
      }
      event "Orbit Plot": Mouse Down {
        n165 = event-data() -> ("Button"=w399:u16)  [unwired: 1 in]
        n166 = Equal?(x=u16 1, y=w399) -> (x = y?=w392:bool)
        n167 = case shown="True" w392 {
          tunnel: w397 -> [w402 w421]
          tunnel: [w402 w420] -> w396
          tunnel: [w401 w418] -> w394
          tunnel: w395 -> [w401 w419]
          tunnel: [_ w413] -> w393
          frame False {
          }
          frame True {
            n168 = Unbundle By Name(w421) -> ("Background Color"=w428:u32, "X Scale.Grid Style"=w412:u16, "X Scale.Major Color"=w411:u32, "X Scale.Minor Color"=w410:u32, "Y Scale.Grid Style"=w407:u16, "Y Scale.Major Color"=w406:u32, "Y Scale.Minor Color"=w405:u32)
            n169 = property on="Orbit Plot" class="XYGraph (strict)"() -> ("BG Color"=w427:u32, "XScale.MajGrdColor"=w426:u32, "XScale.MnrGrdColor"=w425:u32, "YScale.MajGrdColor"=w424:u32, "YScale.MnrGrdColor"=w423:u32)  [unwired: 2 in, 2 out]
            n170 = case shown="0, Default" w412 {
              tunnel: w411 -> [_ w435 w438]
              tunnel: w410 -> [_ _ w437]
              tunnel: [w434 w435 w438] -> w409
              tunnel: [w434 u32 16777216 w437] -> w408
              frame 0, Default {
                w434 = u32 16777216
              }
              frame 1 {
              }
              frame 2 {
              }
            }
            n171 = case shown="0, Default" w407 {
              tunnel: w406 -> [_ w430 w433]
              tunnel: w405 -> [_ _ w432]
              tunnel: [w429 w430 w433] -> w404
              tunnel: [w429 u32 16777216 w432] -> w403
              frame 0, Default {
                w429 = u32 16777216
              }
              frame 1 {
              }
              frame 2 {
              }
            }
            n172 = Bundle("BG Color"=w427, "XScale.MajGrdColor"=w426, "XScale.MnrGrdColor"=w425, "YScale.MajGrdColor"=w424, "YScale.MnrGrdColor"=w423) -> (w422:T14)  [unwired: 1 in]
            n173 = Bundle("Background Color"=w428, "Major Color"=w409, "Minor Color"=w408, "Major Color"=w404, "Minor Color"=w403) -> (w417:T15)  [unwired: 1 in]
            n174 = Not Equal?(x=w417, y=w422) -> (x != y?=w414:cluster{bool, bool, bool, bool, bool})
            n175 = Cluster To Array(cluster=w414) -> (array=w415:bool[])
            n176 = Or Array Elements(Boolean array=w415) -> (logical OR=w416:bool)
            n177 = case shown="True" w416 {
              tunnel: w422 -> [_ w456]
              tunnel: w421 -> [w440 w458]
              tunnel: [w440 w457] -> w420
              tunnel: w419 -> [w439 w455]
              tunnel: [w439 w454] -> w418
              tunnel: w414 -> [_ w446]
              tunnel: [_ w441] -> w413
              frame False {
              }
              frame True {
                w441 = T11[] [enum."[Plot] Grid and BG"] items=["None", "[Axis] Range", "[Plot] Image", "[Plot] Tacho Point", "[Plot] Grid and BG", "[Cursor] Cursor Info", "[Legend] Pair Strings", "[Data] Plot Data", "[Legend] Checkbox", "[Layout] Update", "[Legend] Tree Open", "[Layout] Legend Visible", "[Plot] Data Point", "[Axis] Axis and Label", "[Axis] Format String", "[Cursor] Appearance", "[Cursor] Index", "[Legend] Color", "[Layout] Min Pane Size", "[Data] Legend Strings"]
                n178 = Unbundle(w446) -> (w445:bool, w444:bool, w443:bool)  [unwired: 2 out]
                n179 = Unbundle(w456) -> ("BG Color"=w451:u32, "XScale.MajGrdColor"=w450:u32, "XScale.MnrGrdColor"=w449:u32, "YScale.MajGrdColor"=w448:u32, "YScale.MnrGrdColor"=w447:u32)
                n180 = Or(x=w444, y=w443) -> (x .or. y?=w442:bool)
                n181 = Bundle By Name(cluster=w455, "State Changed?"=TRUE, "Action Name"="Color Changed") -> (w454:T2)
                n182 = case shown="False" w445 {
                  tunnel: w458 -> [w461 w468]
                  tunnel: [w460 w467] -> w457
                  tunnel: w451 -> [w459 _]
                  tunnel: w450 -> [_ w462]
                  tunnel: w449 -> [_ w463]
                  tunnel: w448 -> [_ w465]
                  tunnel: w447 -> [_ w464]
                  tunnel: w442 -> [_ w466]
                  frame True {
                    n183 = Bundle By Name(cluster=w461, "Background Color"=w459) -> (w460:T9)
                  }
                  frame False {
                    n184 = case shown="False" w466 {
                      tunnel: w468 -> [w473 w478]
                      tunnel: [w472 w477] -> w467
                      tunnel: w465 -> [_ w475]
                      tunnel: w464 -> [_ w474]
                      tunnel: w463 -> [w470 _]
                      tunnel: w462 -> [w469 _]
                      frame True {
                        n185 = Bundle By Name(cluster=w473, "X Scale.Major Color"=w469, "X Scale.Minor Color"=w470, "X Scale.Grid Style"=u16 2) -> (w472:T9)
                      }
                      frame False {
                        n186 = Bundle By Name(cluster=w478, "Y Scale.Major Color"=w475, "Y Scale.Minor Color"=w474, "Y Scale.Grid Style"=u16 2 ("X Scale.Grid Style")) -> (w477:T9)
                      }
                    }
                  }
                }
              }
            }
          }
        }
      }
      event "Orbit Plot": Shortcut Menu Selection? (App) {
        n187 = event-data() -> ("ItemTag"=w484:string)  [unwired: 1 in]
        n188 = case shown="\"APP_SC_CLEAR_GRAPH\"" w484 {
          tunnel: w487 -> [w491 w500]
          tunnel: [_ w501] -> w486
          tunnel: [w491 w499] -> w485
          tunnel: w482 -> [w489 _]
          tunnel: [FALSE ("Discard?") TRUE ("Discard?")] -> w483
          tunnel: [w489 T5 [] ("Data In")] -> w481
          tunnel: w480 -> [w488 w494]
          tunnel: [w488 w493] -> w479
          frame Default {
          }
          frame "APP_SC_CLEAR_GRAPH" {
            w492 = string[] [] ("Strings[].row strings []")
            w501 = T11[] [enum."[Data] Plot Data", enum."[Cursor] Cursor Info", enum."[Legend] Pair Strings", enum."[Legend] Checkbox", enum."[Legend] Tree Open"] items=["None", "[Axis] Range", "[Plot] Image", "[Plot] Tacho Point", "[Plot] Grid and BG", "[Cursor] Cursor Info", "[Legend] Pair Strings", "[Data] Plot Data", "[Legend] Checkbox", "[Layout] Update", "[Legend] Tree Open", "[Layout] Legend Visible", "[Plot] Data Point", "[Axis] Axis and Label", "[Axis] Format String", "[Cursor] Appearance", "[Cursor] Index", "[Legend] Color", "[Layout] Min Pane Size", "[Data] Legend Strings"] ("f")
            w495 = TRUE ("State Changed?")
            n189 = Bundle By Name(cluster=w500, "Action Name"="Clear Graph", "Data Changed?"=w495, "State Changed?"=w495) -> (w499:T2)
            n190 = Bundle By Name(cluster=w494, "Strings[].Row Strings []"=w492, "Strings[].Column Strings []"=w492) -> (w493:T9)
          }
        }
        n191 = event-data("Discard?"=w483) -> ()  [unwired: 1 in, 1 out]
      }
      event "Tree": event #0x1e; "Tree": Item Close {
        n192 = event-data() -> ("Tag"=w514:string)  [unwired: 1 in]
        n193 = Unbundle By Name(w510) -> ("Parents Tags"=w515:string[], "Open?"=w513:bool[])
        n194 = Search 1D Array(1D array=w515, element=w514) -> (index of element=w503:i32)  [unwired: 1 in]
        n195 = Index Array(array=w513, index=w503) -> (element=w512:bool)
        n196 = Not(x=w512) -> (.not. x?=w511:bool)
        n197 = Bundle By Name(cluster=w508, "State Changed?"=TRUE, "Action Name"="Item Open") -> (w507:T2)
        n198 = Replace Array Subset(array=w513, new element=w511, index=w503) -> (w502:bool[])
        n199 = Bundle By Name(cluster=w510, "Open?"=w502) -> (w509:T9)
      }
      event "Tree": Mouse Down {
        n200 = event-data() -> ("Coords"=w525:T1)  [unwired: 1 in]
        n201 = Unbundle By Name(w518) -> ("Parents Tags"=w527:string[], "Children Tags"=w526:string[], "Legend Background"=w516:u32)
        n202 = control-ref of="Tree"() -> (w524:refnum<vi>)
        n203 = call <vilib>:"svx_Orbit CheckboxToIndex.vi"("All Children Tags"=w526, "All parents Tags"=w527, "Coords"=w525, "Tree ref in"=w524) -> ("State Changed?"=w523:bool, "index"=w522:cluster{"RowIdx":i32, "ColumnIdx":i32}[])  [unwired: 5 in, 1 out]
        n204 = case shown="True" w523 {
          tunnel: w518 -> [w534 w553]
          tunnel: w522 -> [_ w546]
          tunnel: [w533 w552] -> w521
          tunnel: w520 -> [w532 w551]
          tunnel: [w531 w550] -> w519
          tunnel: [_ w547] -> w517
          tunnel: w516 -> [w535 _]
          frame False {
            w536 = -2 ("Active Cell:Active Column Number")
            n205 = property on="Tree" class="Tree (strict)"("ActiveColNum"=w536, "Active Item Row Number"=w536) -> ("CellBG"=w529:u32)  [unwired: 2 in, 2 out]
            n206 = Equal?(x=w529, y=w535) -> (x = y?=w530:bool)
            n207 = case shown="False" w530 {
              tunnel: w534 -> [w541 w545]
              tunnel: [w540 w545] -> w533
              tunnel: w532 -> [w539 w544]
              tunnel: [w538 w544] -> w531
              tunnel: w529 -> [w537 _]
              frame False {
                n208 = Bundle By Name(cluster=w539, "State Changed?"=TRUE, "Action Name"="Color Change") -> (w538:T2)
                n209 = Bundle By Name(cluster=w541, "Legend Background"=w537) -> (w540:T9)
              }
              frame True {
              }
            }
          }
          frame True {
            w547 = T11[] [enum."[Data] Plot Data", enum."[Axis] Range", enum."[Plot] Image", enum."[Plot] Grid and BG", enum."[Cursor] Cursor Info"] items=["None", "[Axis] Range", "[Plot] Image", "[Plot] Tacho Point", "[Plot] Grid and BG", "[Cursor] Cursor Info", "[Legend] Pair Strings", "[Data] Plot Data", "[Legend] Checkbox", "[Layout] Update", "[Legend] Tree Open", "[Layout] Legend Visible", "[Plot] Data Point", "[Axis] Axis and Label", "[Axis] Format String", "[Cursor] Appearance", "[Cursor] Index", "[Legend] Color", "[Layout] Min Pane Size", "[Data] Legend Strings"]
            n210 = Bundle By Name(cluster=w553, "Index"=w546) -> (w552:T9)
            n211 = Bundle By Name(cluster=w551, "State Changed?"=TRUE, "Action Name"="Selector Changed") -> (w550:T2)
          }
        }
      }
      event "Tree": Shortcut Menu Activation? {
        n212 = event-data() -> ("Coords"=w554:T1)  [unwired: 1 in]
        n213 = local write "Coords"(w554) -> ()
        n214 = event-data("Discard?"=TRUE) -> ()  [unwired: 1 in, 1 out]
      }
      event Shortcut Menu Activation? {
        n215 = event-data() -> ("Coords.Horizontal"=w568:i32, "Coords.Vertical"=w566:i32, "Coords"=w559:T1)  [unwired: 1 in]
        n216 = property on="Orbit Plot" class="XYGraph (strict)"() -> ("Plot Bounds"=w573:T16)  [unwired: 2 in, 2 out]
        n217 = Unbundle By Name(w573) -> ("Right"=w569:i16, "Left"=w567:i16, "Bottom"=w565:i16, "Top"=w564:i16)
        n218 = local write "Coords"(w559) -> ()
        n219 = In Range and Coerce(upper limit=w569, x=w568, lower limit=w567) -> (In Range?=w572:bool)  [unwired: 1 out]
        n220 = In Range and Coerce(upper limit=w565, x=w566, lower limit=w564) -> (In Range?=w571:bool)  [unwired: 1 out]
        n221 = And(x=w572, y=w571) -> (x .and. y?=w570:bool)
        n222 = Not(x=w570) -> (.not. x?=w563:bool)
        n223 = event-data("Discard?"=w563) -> ()  [unwired: 1 in, 1 out]
      }
      event Mouse Down? {
        n224 = event-data() -> ("Button"=w578:u16, "Mods"=w579:cluster{"Double Click":bool, "Menu Key":bool}, "PlatMods"=w576:T17, "Coords"=w574:T1)  [unwired: 1 in]
        n225 = case shown="1" w578 {
          tunnel: w579 -> [w587 w591]
          tunnel: [w590 w591] -> w577
          tunnel: w574 -> [w589 _]
          frame 1 {
            n226 = local read "Coords"() -> (w588:T1)
            n227 = Unbundle By Name(w587) -> ("Double Click"=w585:bool)
            n228 = Equal?(x=w589, y=w588) -> (x = y?=w586:bool)
            n229 = Select(t=FALSE ("Double Click"), s=w586, f=w585) -> (s? t:f=w583:bool)
            n230 = Bundle By Name(cluster=w587, "Double Click"=w583) -> (w590:cluster{"Double Click":bool, "Menu Key":bool})
          }
          frame 0, Default {
          }
        }
        n231 = event-data("Button"=w578, "Mods"=w577, "PlatMods"=w576, "Discard?"=FALSE) -> ()  [unwired: 1 in, 1 out]
      }
    }
    n232 = flat-sequence {
      tunnel: w22 -> [w38]
      tunnel: w21 -> [w37]
      tunnel: w20 -> [w36]
      tunnel: w19 -> [w35]
      tunnel: [w30] -> w14
      tunnel: w10 -> [w28]
      tunnel: w9 -> [w27]
      tunnel: [w27] -> w8
      tunnel: w14 -> [w50]
      tunnel: w13 -> [w51]
      tunnel: w12 -> [w48]
      tunnel: [w47] -> w11
      tunnel: w8 -> [w45]
      frame #0 {
        n233 = case shown="False" w28 {
          tunnel: w36 -> [w43 w44]
          tunnel: [w42 w44] -> w29
          tunnel: w27 -> [w41 _]
          frame False {
            n234 = Unbundle By Name(w41) -> ("Container Bounds"=w40:T10, "Legend Width"=w39:u32)
            n235 = Bundle By Name(cluster=w43, "Container Bounds"=w40, "Legend Width"=w39) -> (w42:T9)
          }
          frame True {
          }
        }
        n236 = control-ref of="Orbit Plot"() -> (w31:refnum<vi>)
        n237 = control-ref of="Tree"() -> (w32:refnum<vi>)
        n238 = control-ref of="Cursor Info"() -> (w33:refnum<vi>)
        n239 = control-ref of="This VI"() -> (w34:refnum<vi>)
        n240 = call <vilib>:"svx_Orbit Exec Commands.vi"("Display State In"=w29, "Data In"=w37, "Commands"=w35, "Container"=w38, "Facade VI"=w34, "Cursor Info"=w33, "Tree"=w32, "Orbit Plot"=w31) -> ("Display State Out"=w30:T9)  [unwired: 3 in]
      }
      frame #1 {
        n241 = To Variant(anything=w45) -> (Variant=w46:variant)
        n242 = Dequeue Element(queue=w51) -> (queue out=w49:refnum<queue>)  [unwired: 2 in, 3 out]
        n243 = Enqueue Element(queue=w49, element=w50) -> ()  [unwired: 2 in, 3 out]
        n244 = Bundle By Name(cluster=w48, "Old State"=w46) -> (w47:T3)
      }
    }
    n245 = Unbundle By Name(w23) -> ("Refnum"=w22:refnum<vi>)
  }
  "Display State Out" <- w4
  "Data Out" <- w7
  "Action" <- w2
